vi "1 BIT Register.vi"(1 "Clock":bool, 2 "Hold":bool, 3 "Data":bool) -> (0 "Q":bool)   [LabVIEW 2012]
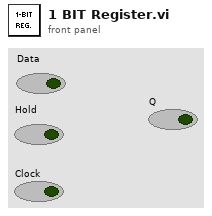
[diagram p1: front panel]
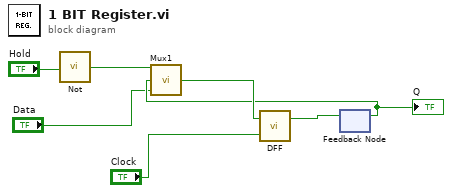
[diagram p0: block diagram]
diagram:
  n1 = call "Not.vi"("In"="Hold") -> ("Out"=w2:bool)
  n2 = feedback #1() -> (w5:bool)  [unwired: 1 in]
  "Q" <- w5
  n3 = call "Mux1.vi"("B"="Data", "A"=w5, "s0"=w2) -> ("z"=w7:bool)
  n4 = call "DFF.vi"("Clock"="Clock", "D"=w7) -> ("Q"=w6:bool)  [unwired: 1 out]
  n5 = feedback-in #1(w6) -> ()
